vi "Write Write Directory.vi"(8 "error in (no error)":errorcluster, 10 "write directory":path, 11 "shared memory configuration in":refnum<class "shared memory configuration.lvclass">) -> (0 "error out":errorcluster, 3 "shared memory configuration out":refnum<class "shared memory configuration.lvclass">)   [LabVIEW 2013, in "shared memory configuration.lvclass"]
uses:
  shared memory configuration.lvclass
  shared memory configuration.lvclass/shared memory configuration.ctl
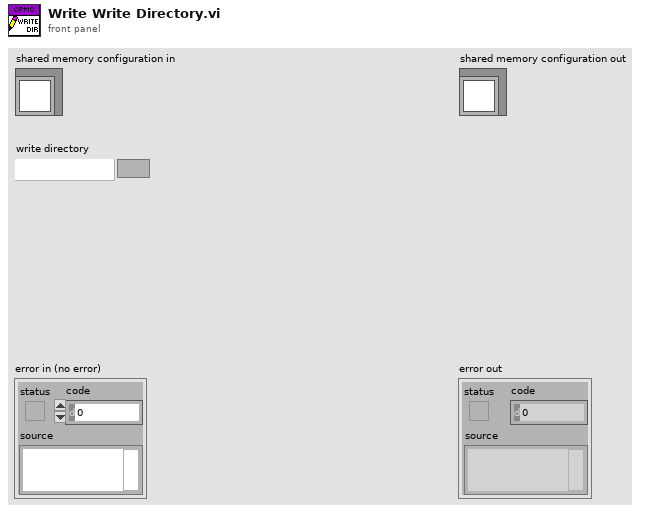
[diagram p1: front panel]
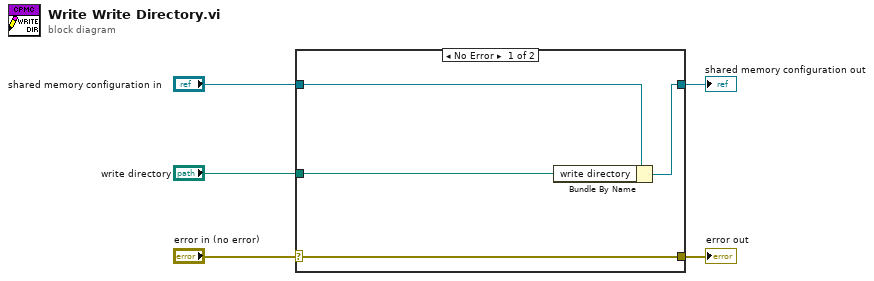
[diagram p0: block diagram]
diagram:
  n1 = case shown="No Error" "error in (no error)" {
    selector: "error in (no error)" -> [w9 w10]
    tunnel: [w9 w10] -> w4
    tunnel: [w7 w11] -> w2
    tunnel: "shared memory configuration in" -> [w8 w11]
    tunnel: "write directory" -> [w6 _]
    frame No Error {
      n2 = Bundle By Name(cluster=w8, "write directory"=w6) -> (w7:refnum<class "shared memory configuration.lvclass">)
    }
    frame Error {
    }
  }
  "error out" <- w4
  "shared memory configuration out" <- w2
